vi "Stop.vi"(8 "error in (no error)":errorcluster, 11 "Motor-Maxon in":refnum<class "Motor-Maxon.lvclass">) -> (0 "error out":errorcluster, 3 "Motor-Maxon out":refnum<class "Motor-Maxon.lvclass">)   [LabVIEW 2013, in "PowderDeposition.lvlib" / "Motor-Maxon.lvclass"]
uses:
  Motor-Maxon.lvclass
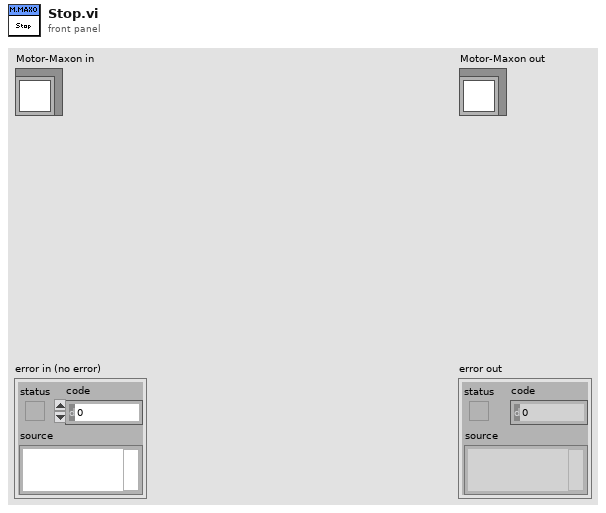
[diagram p1: front panel]
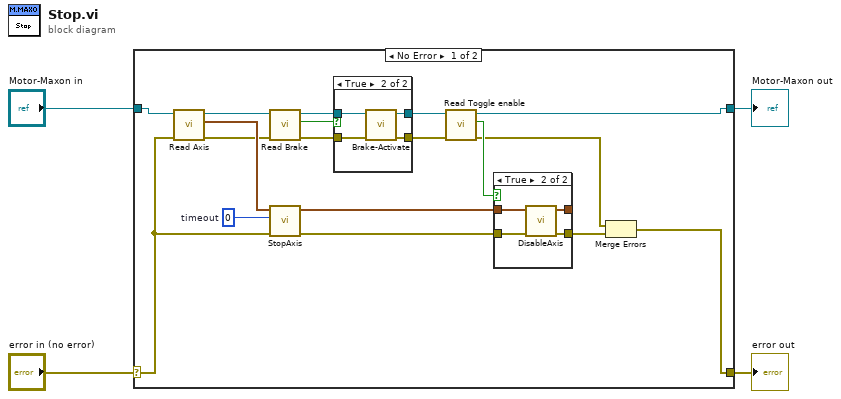
[diagram p0: block diagram]
diagram:
  n1 = case shown="No Error" "error in (no error)" {
    selector: "error in (no error)" -> [w18 w36]
    tunnel: [w5 w36] -> w3
    tunnel: [w7 w35] -> w1
    tunnel: "Motor-Maxon in" -> [w21 w35]
    frame No Error {
      w19 = u32 0  # timeout
      n2 = call-dynamic "Read Axis.vi"("error in (no error)"=w18, "Motor-Maxon in"=w21) -> ("error out"=w13:errorcluster, "Axis"=w20:cluster{"keyHandle":u32, "nodeID":u16}, "Motor-Maxon out"=w17:refnum<class "Motor-Maxon.lvclass">)  [unwired: 7 in]
      n3 = call-dynamic "Read Brake.vi"("error in (no error)"=w13, "Motor-Maxon in"=w17) -> ("error out"=w14:errorcluster, "Brake"=w16:bool, "Motor-Maxon out"=w15:refnum<class "Motor-Maxon.lvclass">)  [unwired: 7 in]
      n4 = call <instrlib>:"StopAxis.vi"("error in (no error)"=w18, "timeout"=w19, "axis in"=w20) -> ("error out"=w9:errorcluster, "axis out"=w10:cluster{"keyHandle":u32, "nodeId":u16})  [unwired: 3 in]
      n5 = case shown="True" w16 {
        tunnel: w15 -> [w24 w28]
        tunnel: w14 -> [w23 w27]
        tunnel: [w24 w26] -> w12
        tunnel: [w23 w25] -> w11
        frame False {
        }
        frame True {
          n6 = call-dynamic "Brake-Activate.vi"("error in (no error)"=w27, "Motor-Maxon in"=w28) -> ("error out"=w25:errorcluster, "Motor-Maxon out"=w26:refnum<class "Motor-Maxon.lvclass">)  [unwired: 8 in]
        }
      }
      n7 = call-dynamic "Read Toggle enable.vi"("error in (no error)"=w11, "Motor-Maxon in"=w12) -> ("error out"=w6:errorcluster, "Toggle enable"=w22:bool, "Motor-Maxon out"=w7:refnum<class "Motor-Maxon.lvclass">)  [unwired: 7 in]
      n8 = case shown="True" w22 {
        tunnel: w10 -> [w30 w33]
        tunnel: w9 -> [w29 w34]
        tunnel: [w30 w32] -> _
        tunnel: [w29 w31] -> w8
        frame False {
        }
        frame True {
          n9 = call <instrlib>:"DisableAxis.vi"("error in (no error)"=w34, "axis in"=w33) -> ("error out"=w31:errorcluster, "axis out"=w32:cluster{"keyHandle":u32, "nodeId":u16})  [unwired: 4 in]
        }
      }
      n10 = Merge Errors(w6, w8) -> (w5:errorcluster)
    }
    frame Error {
    }
  }
  "error out" <- w3
  "Motor-Maxon out" <- w1
